vi "HandleFIFOsetting_new.vi"(8 "timed out":bool, 11 "Value":u64) -> ()   [LabVIEW 2013]
uses:
  <vilib>/rvi/DataTransferAndStorage/Register/Emulation/niFpgaRegisterEmulationFpgaImpl.vi
  <instcachedir>/0/niFpgaRegisterEmulationFpgaImpl_DCF4BC0110594B98B44A971D60CEEC4D.lvgen/niFpgaRegisterEmulationFpgaImpl_DCF4BC0110594B98B44A971D60CEEC4D_003.vi
  <vilib>/rvi/DataTransferAndStorage/Container/Common/niFpgaContainerGetUniqueNameForEmu.vi
  <instcachedir>/0/niFpgaRegisterEmulationFpgaImpl_DCF4BC0110594B98B44A971D60CEEC4D.lvgen/niFpgaRegisterEmulationFpgaImpl_DCF4BC0110594B98B44A971D60CEEC4D_016.vi
  <instcachedir>/0/niFpgaRegisterEmulationFpgaImpl_DCF4BC0110594B98B44A971D60CEEC4D.lvgen/niFpgaRegisterEmulationFpgaImpl_DCF4BC0110594B98B44A971D60CEEC4D_015.vi
  <instcachedir>/0/niFpgaRegisterEmulationFpgaImpl_DCF4BC0110594B98B44A971D60CEEC4D.lvgen/niFpgaRegisterEmulationFpgaImpl_DCF4BC0110594B98B44A971D60CEEC4D_014.vi
  <instcachedir>/0/niFpgaRegisterEmulationFpgaImpl_DCF4BC0110594B98B44A971D60CEEC4D.lvgen/niFpgaRegisterEmulationFpgaImpl_DCF4BC0110594B98B44A971D60CEEC4D_013.vi
  <instcachedir>/0/niFpgaRegisterEmulationFpgaImpl_DCF4BC0110594B98B44A971D60CEEC4D.lvgen/niFpgaRegisterEmulationFpgaImpl_DCF4BC0110594B98B44A971D60CEEC4D_012.vi
  <instcachedir>/0/niFpgaRegisterEmulationFpgaImpl_DCF4BC0110594B98B44A971D60CEEC4D.lvgen/niFpgaRegisterEmulationFpgaImpl_DCF4BC0110594B98B44A971D60CEEC4D_011.vi
  <instcachedir>/0/niFpgaRegisterEmulationFpgaImpl_DCF4BC0110594B98B44A971D60CEEC4D.lvgen/niFpgaRegisterEmulationFpgaImpl_DCF4BC0110594B98B44A971D60CEEC4D_010.vi
  <instcachedir>/0/niFpgaRegisterEmulationFpgaImpl_DCF4BC0110594B98B44A971D60CEEC4D.lvgen/niFpgaRegisterEmulationFpgaImpl_DCF4BC0110594B98B44A971D60CEEC4D_008.vi
  <instcachedir>/0/niFpgaRegisterEmulationFpgaImpl_DCF4BC0110594B98B44A971D60CEEC4D.lvgen/niFpgaRegisterEmulationFpgaImpl_DCF4BC0110594B98B44A971D60CEEC4D_007.vi
  <instcachedir>/0/niFpgaRegisterEmulationFpgaImpl_DCF4BC0110594B98B44A971D60CEEC4D.lvgen/niFpgaRegisterEmulationFpgaImpl_DCF4BC0110594B98B44A971D60CEEC4D_009.vi
  <instcachedir>/0/niFpgaRegisterEmulationFpgaImpl_DCF4BC0110594B98B44A971D60CEEC4D.lvgen/niFpgaRegisterEmulationFpgaImpl_DCF4BC0110594B98B44A971D60CEEC4D_020.vi
  <instcachedir>/0/niFpgaRegisterEmulationFpgaImpl_DCF4BC0110594B98B44A971D60CEEC4D.lvgen/niFpgaRegisterEmulationFpgaImpl_DCF4BC0110594B98B44A971D60CEEC4D_021.vi
  <vilib>/rvi/DataTransferAndStorage/Container/XNode/niFpgaContainer.xnode
  <vilib>/rvi/DataTransferAndStorage/Register/Emulation/niFpgaRegisterEmulation.vi
  <vilib>/rvi/FXPMathLib/FxpInterpret/XNode/nifxpmath_Interpret.xnode
  fpga_settings.ctl
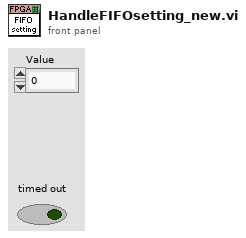
[diagram p1: front panel]
types:
  T1 = typedef "fpga_settings.ctl" = enum16{"Feedback Enable", "New FIR coeffs", "FIR shift", "Enable filter", "Set Downsample", "Downsample", "CIC Gain", "Record length", "Trigger samples", "Quiet time", "a_am", "b_am", "Use fixed delay", "fixed sin_fi", "fixed cos_fi", "Ki*Tau", "Kp", "Kd_Tau", "Fi_start", "Fi_delta", "DC_offs 0", "DC_offs 1", "DC_offs 2", "DC_offs 3", "Ki*Tau am", "Kp am", "Kd_Tau am", "Feedback AM"}
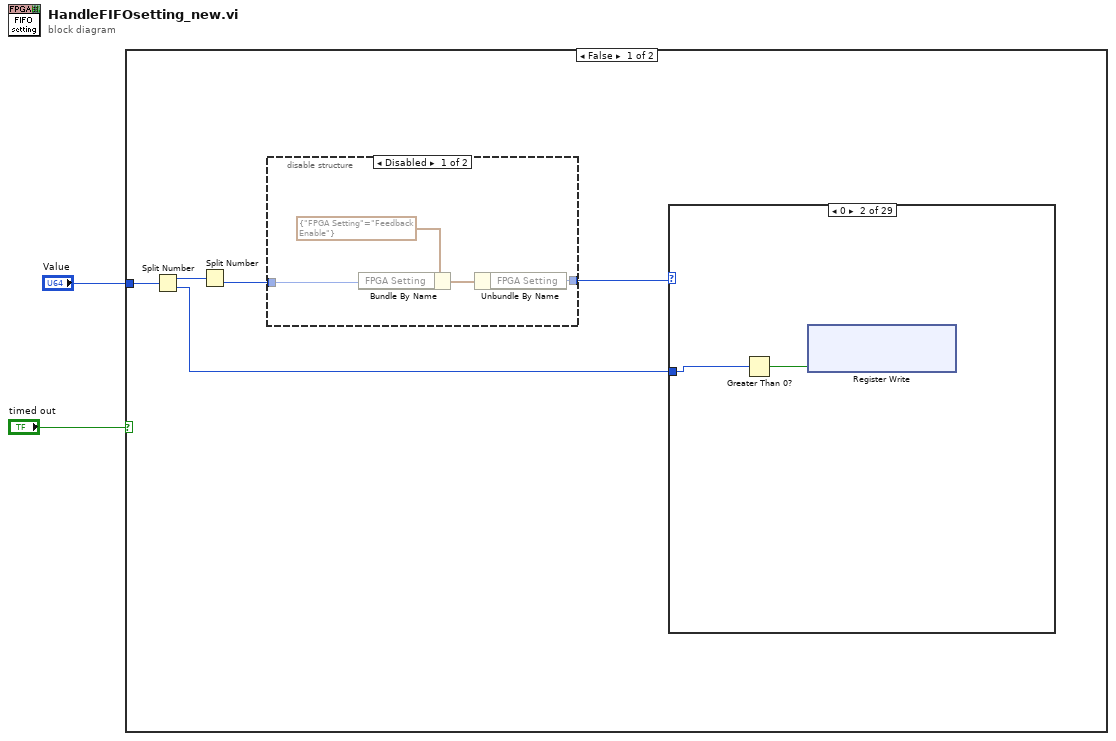
[diagram p0: block diagram]
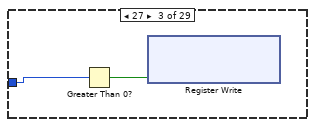
[diagram p4: hidden frame]
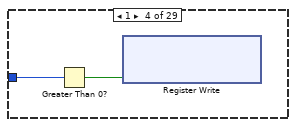
[diagram p5: hidden frame]
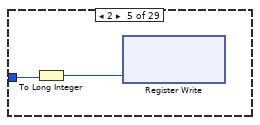
[diagram p6: hidden frame]
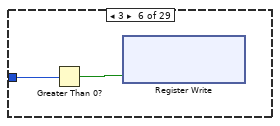
[diagram p7: hidden frame]
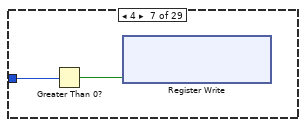
[diagram p8: hidden frame]
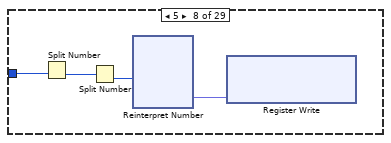
[diagram p9: hidden frame]
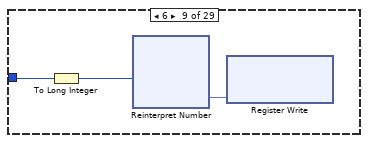
[diagram p10: hidden frame]
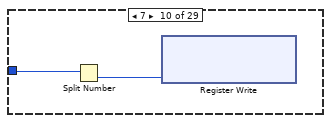
[diagram p11: hidden frame]
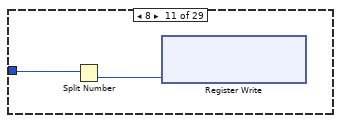
[diagram p12: hidden frame]
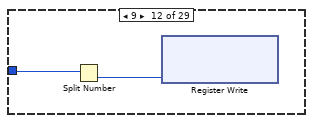
[diagram p13: hidden frame]
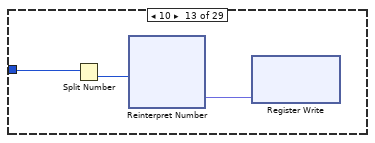
[diagram p14: hidden frame]
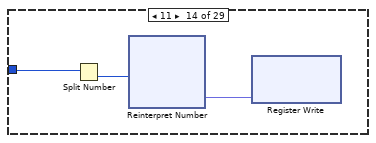
[diagram p15: hidden frame]
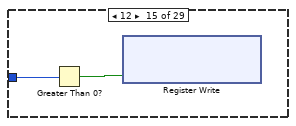
[diagram p16: hidden frame]
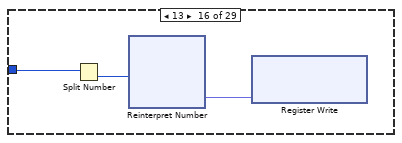
[diagram p17: hidden frame]
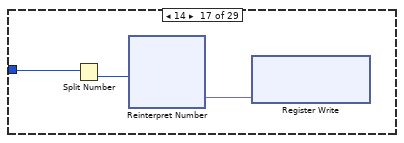
[diagram p18: hidden frame]
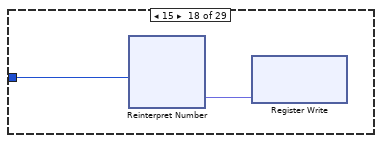
[diagram p19: hidden frame]
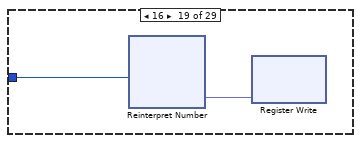
[diagram p20: hidden frame]
diagram:
  n1 = case shown="False" "timed out" {
    tunnel: "Value" -> [w7 _]
    frame False {
      n2 = Split Number(x=w7) -> (hi(x)=w6:u32, lo(x)=w3:u32)
      n3 = Split Number(x=w6) -> (lo(x)=w5:u16)  [unwired: 1 out]
      n4 = disable-structure shown="Disabled" {
        disable-tunnel: [w9 w12] -> w4
        disable-tunnel: w5 -> [w8 w12]
        frame Disabled {
          n5 = Bundle By Name(cluster=cluster{"FPGA Setting":T1} {"FPGA Setting"=enum."Feedback Enable"}, "FPGA Setting"=w8) -> (w10:cluster{"FPGA Setting":T1})
          n6 = Unbundle By Name(w10) -> ("FPGA Setting"=w9:T1)
        }
        frame Enabled {
        }
      }
      n7 = case shown="0" w4 {
        tunnel: w3 -> [_ w13 w15 w18 w20 w22 w24 w28 w30 w33 w35 w37 w40 w43 w45 w48 w51 w52 w54 w56 w58 w60 w64 w67 w70 w73 w74 w76 w78]
        frame Default {
        }
        frame 0 {
          n8 = Greater Than 0?(x=w13) -> (x > 0?=w14:bool)
          n9 = xnode ("Register Write")("Data"=w14) -> ()  [unwired: 1 in, 1 out]
        }
        frame 27 {
          n10 = Greater Than 0?(x=w15) -> (x > 0?=w16:bool)
          n11 = xnode ("Register Write")("Data"=w16) -> ()  [unwired: 1 in, 1 out]
        }
        frame 1 {
          n12 = Greater Than 0?(x=w18) -> (x > 0?=w17:bool)
          n13 = xnode ("Register Write")("Data"=w17) -> ()  [unwired: 1 in, 1 out]
        }
        frame 2 {
          n14 = To Long Integer(number=w20) -> (32bit integer=w19:i32)
          n15 = xnode ("Register Write")("Data"=w19) -> ()  [unwired: 1 in, 1 out]
        }
        frame 3 {
          n16 = Greater Than 0?(x=w22) -> (x > 0?=w21:bool)
          n17 = xnode ("Register Write")("Data"=w21) -> ()  [unwired: 1 in, 1 out]
        }
        frame 4 {
          n18 = Greater Than 0?(x=w24) -> (x > 0?=w23:bool)
          n19 = xnode ("Register Write")("Data"=w23) -> ()  [unwired: 1 in, 1 out]
        }
        frame 5 {
          n20 = Split Number(x=w28) -> (lo(x)=w27:u16)  [unwired: 1 out]
          n21 = Split Number(x=w27) -> (lo(x)=w26:u8)  [unwired: 1 out]
          n22 = xnode "Reinterpret Number"("x"=w26) -> ("y"=w25:fxp<+,8,8>)
          n23 = xnode ("Register Write")("Data"=w25) -> ()  [unwired: 1 in, 1 out]
        }
        frame 6 {
          n24 = To Long Integer(number=w30) -> (32bit integer=w29:i32)
          n25 = xnode "Reinterpret Number"("x"=w29) -> ("y"=w31:fxp<+/-,32,1>)
          n26 = xnode ("Register Write")("Data"=w31) -> ()  [unwired: 1 in, 1 out]
        }
        frame 7 {
          n27 = Split Number(x=w33) -> (lo(x)=w32:u16)  [unwired: 1 out]
          n28 = xnode ("Register Write")("Data"=w32) -> ()  [unwired: 1 in, 1 out]
        }
        frame 8 {
          n29 = Split Number(x=w35) -> (lo(x)=w34:u16)  [unwired: 1 out]
          n30 = xnode ("Register Write")("Data"=w34) -> ()  [unwired: 1 in, 1 out]
        }
        frame 9 {
          n31 = Split Number(x=w37) -> (lo(x)=w36:u16)  [unwired: 1 out]
          n32 = xnode ("Register Write")("Data"=w36) -> ()  [unwired: 1 in, 1 out]
        }
        frame 10 {
          n33 = Split Number(x=w40) -> (lo(x)=w39:u16)  [unwired: 1 out]
          n34 = xnode "Reinterpret Number"("x"=w39) -> ("y"=w38:fxp<+/-,16,2>)
          n35 = xnode ("Register Write")("Data"=w38) -> ()  [unwired: 1 in, 1 out]
        }
        frame 11 {
          n36 = Split Number(x=w43) -> (lo(x)=w42:u16)  [unwired: 1 out]
          n37 = xnode "Reinterpret Number"("x"=w42) -> ("y"=w41:fxp<+/-,16,2>)
          n38 = xnode ("Register Write")("Data"=w41) -> ()  [unwired: 1 in, 1 out]
        }
        frame 12 {
          n39 = Greater Than 0?(x=w45) -> (x > 0?=w44:bool)
          n40 = xnode ("Register Write")("Data"=w44) -> ()  [unwired: 1 in, 1 out]
        }
        frame 13 {
          n41 = Split Number(x=w48) -> (lo(x)=w47:u16)  [unwired: 1 out]
          n42 = xnode "Reinterpret Number"("x"=w47) -> ("y"=w46:fxp<+/-,16,0>)
          n43 = xnode ("Register Write")("Data"=w46) -> ()  [unwired: 1 in, 1 out]
        }
        frame 14 {
          n44 = Split Number(x=w51) -> (lo(x)=w50:u16)  [unwired: 1 out]
          n45 = xnode "Reinterpret Number"("x"=w50) -> ("y"=w49:fxp<+/-,16,0>)
          n46 = xnode ("Register Write")("Data"=w49) -> ()  [unwired: 1 in, 1 out]
        }
        frame 15 {
          n47 = xnode "Reinterpret Number"("x"=w52) -> ("y"=w53:fxp<+/-,32,4>)
          n48 = xnode ("Register Write")("Data"=w53) -> ()  [unwired: 1 in, 1 out]
        }
        frame 16 {
          n49 = xnode "Reinterpret Number"("x"=w54) -> ("y"=w55:fxp<+/-,32,4>)
          n50 = xnode ("Register Write")("Data"=w55) -> ()  [unwired: 1 in, 1 out]
        }
        frame 17 {
          n51 = xnode "Reinterpret Number"("x"=w56) -> ("y"=w57:fxp<+/-,32,4>)
          n52 = xnode ("Register Write")("Data"=w57) -> ()  [unwired: 1 in, 1 out]
        }
        frame 18 {
          n53 = xnode "Reinterpret Number"("x"=w58) -> ("y"=w59:fxp<+/-,32,4>)
          n54 = xnode ("Register Write")("Data"=w59) -> ()  [unwired: 1 in, 1 out]
        }
        frame 19 {
          n55 = xnode "Reinterpret Number"("x"=w60) -> ("y"=w61:fxp<+/-,32,4>)
          n56 = xnode ("Register Write")("Data"=w61) -> ()  [unwired: 1 in, 1 out]
        }
        frame 20 {
          n57 = Split Number(x=w64) -> (lo(x)=w63:u16)  [unwired: 1 out]
          n58 = xnode "Reinterpret Number"("x"=w63) -> ("y"=w62:fxp<+/-,16,14>)
          n59 = xnode ("Register Write")("Data"=w62) -> ()  [unwired: 1 in, 1 out]
        }
        frame 21 {
          n60 = Split Number(x=w67) -> (lo(x)=w66:u16)  [unwired: 1 out]
          n61 = xnode "Reinterpret Number"("x"=w66) -> ("y"=w65:fxp<+/-,16,14>)
          n62 = xnode ("Register Write")("Data"=w65) -> ()  [unwired: 1 in, 1 out]
        }
        frame 22 {
          n63 = Split Number(x=w70) -> (lo(x)=w69:u16)  [unwired: 1 out]
          n64 = xnode "Reinterpret Number"("x"=w69) -> ("y"=w68:fxp<+/-,16,14>)
          n65 = xnode ("Register Write")("Data"=w68) -> ()  [unwired: 1 in, 1 out]
        }
        frame 23 {
          n66 = Split Number(x=w73) -> (lo(x)=w72:u16)  [unwired: 1 out]
          n67 = xnode "Reinterpret Number"("x"=w72) -> ("y"=w71:fxp<+/-,16,14>)
          n68 = xnode ("Register Write")("Data"=w71) -> ()  [unwired: 1 in, 1 out]
        }
        frame 24 {
          n69 = xnode "Reinterpret Number"("x"=w74) -> ("y"=w75:fxp<+/-,32,6>)
          n70 = xnode ("Register Write")("Data"=w75) -> ()  [unwired: 1 in, 1 out]
        }
        frame 25 {
          n71 = xnode "Reinterpret Number"("x"=w76) -> ("y"=w77:fxp<+/-,32,6>)
          n72 = xnode ("Register Write")("Data"=w77) -> ()  [unwired: 1 in, 1 out]
        }
        frame 26 {
          n73 = xnode "Reinterpret Number"("x"=w78) -> ("y"=w79:fxp<+/-,32,6>)
          n74 = xnode ("Register Write")("Data"=w79) -> ()  [unwired: 1 in, 1 out]
        }
      }
    }
    frame True {
    }
  }
